vi "Error Dialog.vi"(0 "Clear Error?":bool, 11 "error in":errorcluster) -> (6 "Shutdown":bool, 15 "error out":errorcluster)   [LabVIEW 2016]
doc: "Generates a custom popup dialog. Displays the <b>error in</b> information, including error <b>code</b> and <b>source</b>.\n\nOptionally <b>Clears Error</b> before passing <b>error out</b> to upper-level diagram."
uses:
  <vilib>/Utility/error.llb/DialogType.ctl
panel:
  in  "Continue":bool
  in  "Quit":bool
  out "Error Code":string
  out "Display Source":string
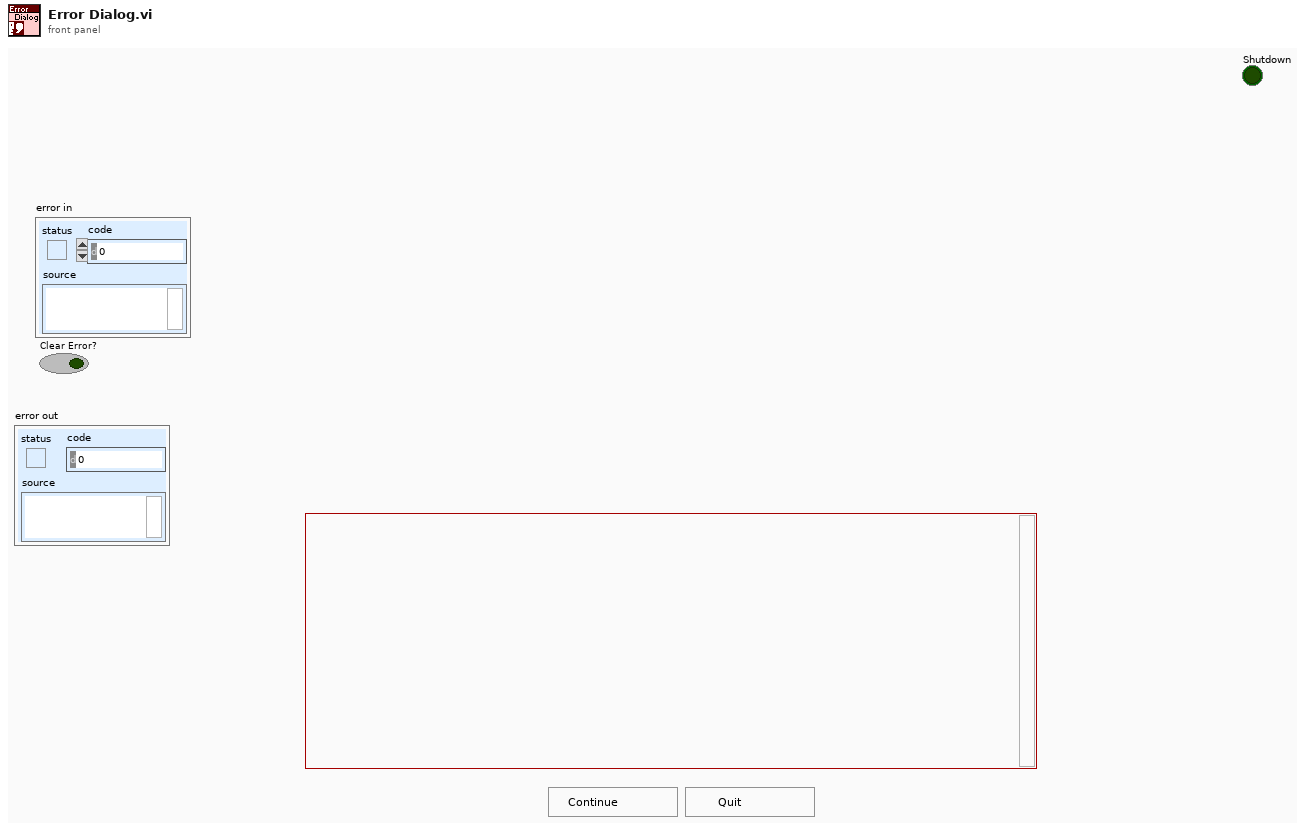
[diagram p1: front panel]
types:
  T1 = typedef "DialogType.ctl" = u16
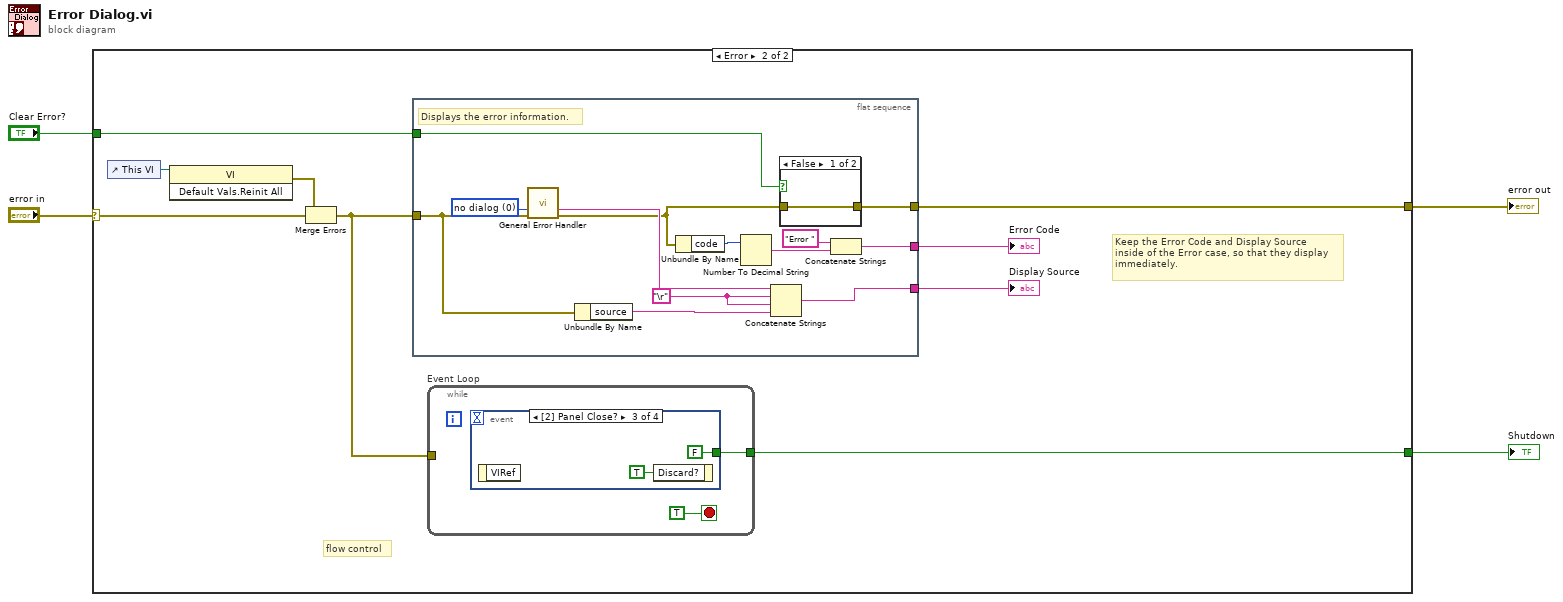
[diagram p0: block diagram]
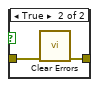
[diagram p3: hidden frame]
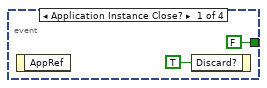
[diagram p4: hidden frame]
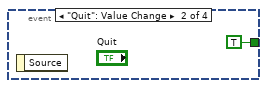
[diagram p5: hidden frame]
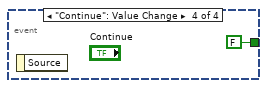
[diagram p6: hidden frame]
diagram:
  n1 = case shown="Error" "error in" {
    selector: "error in" -> [w5 w10]
    tunnel: [w5 w14] -> w4
    tunnel: "Clear Error?" -> [_ w13]
    tunnel: [_ w8] -> w2
    frame No Error {
    }
    frame Error {
      # "flow control"
      # "Keep the Error Code and Display Source\ninside of the Error case, so that they display\nimmediately."
      n2 = control-ref of="This VI"() -> (w7:refnum<vi>)
      n3 = invoke class="VI" method="Default Vals.Reinit All"(reference=w7) -> (error out=w6:errorcluster)  [unwired: 2 in, 2 out]
      n4 = Merge Errors(w6, w10) -> (w9:errorcluster)
      n5 = flat-sequence {
        tunnel: w9 -> [w16]
        tunnel: [w20] -> w14
        tunnel: [w25] -> w12
        tunnel: [w18] -> w11
        tunnel: w13 -> [w19]
        frame #0 {
          w17 = "\r"
          w23 = T1 0 items=["no dialog", "OK message", "continue or stop message", "OK message + warnings", "continue/stop + warnings"] ("type of dialog (OK msg:1)")
          # "Displays the error information."
          n6 = call <vilib>:"General Error Handler.vi"("type of dialog (OK msg:1)"=w23, "error in (no error)"=w16) -> ("message"=w22:string, "error out"=w21:errorcluster)  [unwired: 9 in, 3 out]
          n7 = Unbundle By Name(w16) -> ("source"=w15:string)
          n8 = Unbundle By Name(w21) -> ("code"=w24:i32)
          n9 = Number To Decimal String(number=w24) -> (decimal integer string=w26:string)  [unwired: 1 in]
          n10 = Concatenate Strings(w22, w17, w17, w15) -> (w18:string)
          n11 = case shown="False" w19 {
            tunnel: w21 -> [w28 w30]
            tunnel: [w28 w29] -> w20
            frame False {
            }
            frame True {
              n12 = call <vilib>:"Clear Errors.vi"("error in (no error)"=w30) -> ("error out"=w29:errorcluster)  [unwired: 5 in, 1 out]
            }
          }
          n13 = Concatenate Strings("Error " ("string"), w26) -> (w25:string)
        }
      }
      n14 = while "Event Loop" {
        tunnel: [w31] -> w8
        tunnel: w9 -> [_]
        stop <- TRUE stop-if-true
        n15 = event shown="[2] Panel Close?" {
          selector: _ -> [_ _ _ _]
          dyn-events: _ -> [_ _ _ _]
          timeout: _ -> [_ _ _ _]
          tunnel: [FALSE ("Discard?") TRUE ("Discard?") FALSE ("Discard?") FALSE ("Discard?")] -> w31
          event Application Instance Close? {
            n16 = event-data() -> ()  [unwired: 1 in, 1 out]
            n17 = event-data("Discard?"=TRUE) -> ()  [unwired: 1 in, 1 out]
          }
          event "Quit": Value Change {
            n18 = event-data() -> ()  [unwired: 1 in, 1 out]
          }
          event Panel Close? {
            n19 = event-data() -> ()  [unwired: 1 in, 1 out]
            n20 = event-data("Discard?"=TRUE) -> ()  [unwired: 1 in, 1 out]
          }
          event "Continue": Value Change {
            n21 = event-data() -> ()  [unwired: 1 in, 1 out]
          }
        }
      }
      "Error Code" <- w12
      "Display Source" <- w11
    }
  }
  "error out" <- w4
  "Shutdown" <- w2
